vi "CRYAPI LOAD.vi"(4 "sTitle":string, 6 "sOption":string, 8 "sData":string, 9 "nData":i32, 10 "pSPRef":refnum<vi>, 11 "sAction":string) -> (0 "nData_Out":i32, 1 "tWindow_Out":T1, 2 "pVIRef_Out":refnum<vi>, 3 "pSPRef_Out":refnum<vi>)   [LabVIEW 2013]
uses:
  CRYMain Sub Window Global.vi
  DataView/VIEW/CRYView Global.vi
  CRYDocument/CRYReport Global.vi
  CRYProject/CRYProject Editor Global.vi
  CRYStepSetup/CRYStepSetup Global.vi
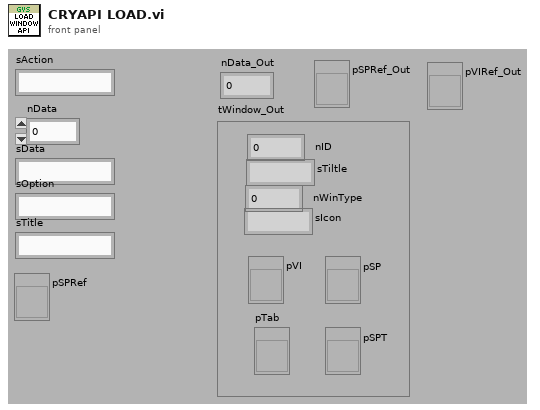
[diagram p1: front panel]
types:
  T1 = cluster{"nID":i32, "sTiltle":string, "pVI":refnum<vi>, "pSP":refnum<vi>, "pTab":refnum<vi>, "pSPT":refnum<vi>, "nWinType":i32, "sIcon":string}
  T2 = cluster{"sAction":string, "sType":string, "sQueueName":string, "sGraphName":string, "sData":string, "nData":i32, "pVIRef":refnum<vi>, "pSPRef":refnum<vi>}
  T3 = typedef "CRYTS.ctl" = cluster{"No.TS":u16, "TS File Path":path, "TS Name":string, "EditStepName":string, "Steps":T4[], "New State":bool, "Change State":bool, "Flattened CurveLib Data":string, "Document Data":string, "EditStepNo":u16, "Operator Start File":string, "Sequence Type":string, "Sequence Language":string}
  T4 = typedef "CRYStep.ctl" = cluster{"No.VI":i32, "Category":string, "StepName":string, "Seq setup flattened":string, "Comment":string, "Steps config.":bool[], "Jump config":i32[], "Start":dbl, "Increment":dbl, "Name":string, "Unit":string, "Y data":u16, "Y prefix":string, "Y dB ref":dbl, "Y unit":string, "Repeat State Array":cluster{"Start":dbl, "Increment":dbl, "Count":i32, "Num":i32}[]}
  T5 = cluster{"CLOSE_HIDE":i32, "CLOSE_CLOSE":i32, "DOCK_ENABLE":i32, "DOCK_DISABLE":i32, "FOCUS_SHOW":i32, "FOCUS_HIDE":i32}
  T6 = cluster{"sStepName":string, "nStepVINo":i32, "nStepVINoDisplay":i32}
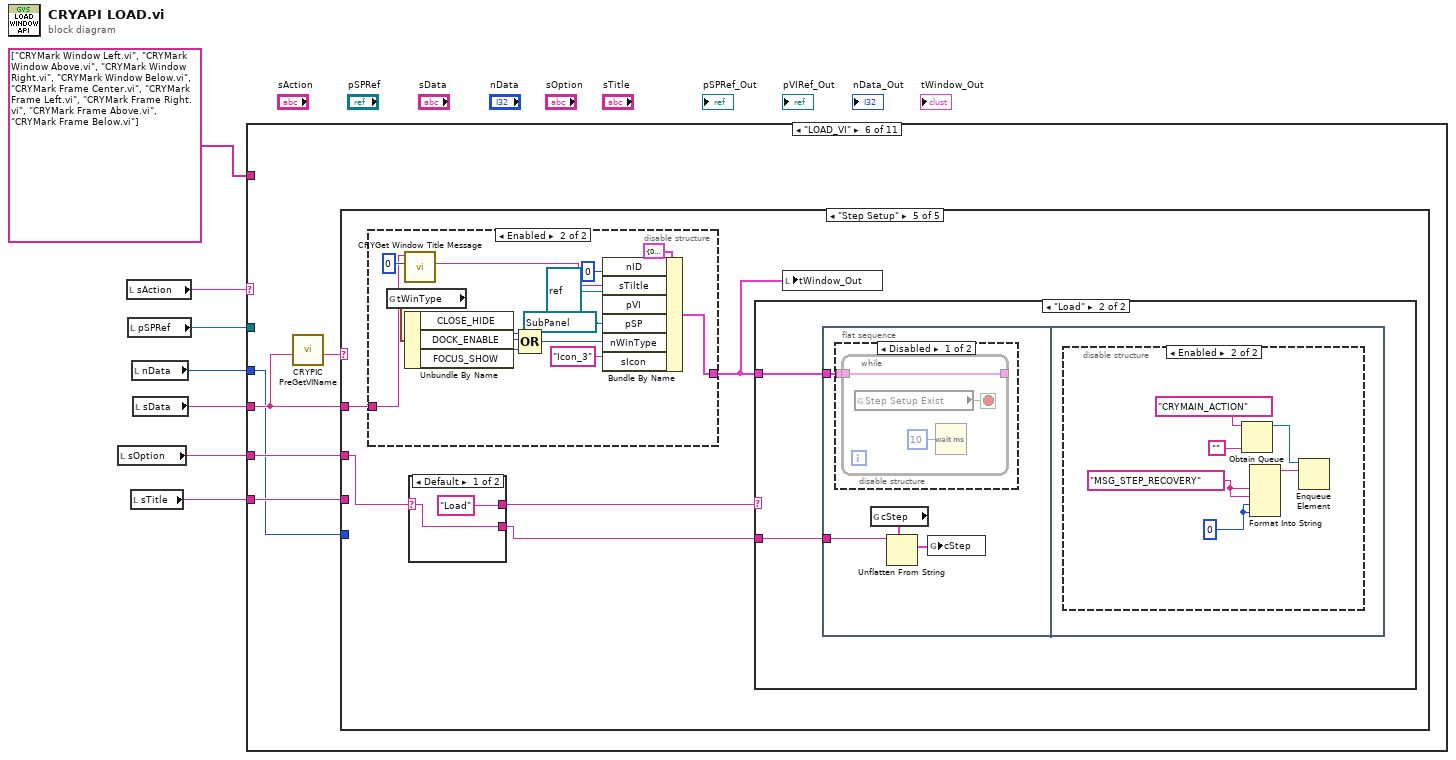
[diagram p0: block diagram]
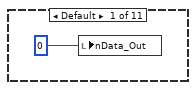
[diagram p2: hidden frame]
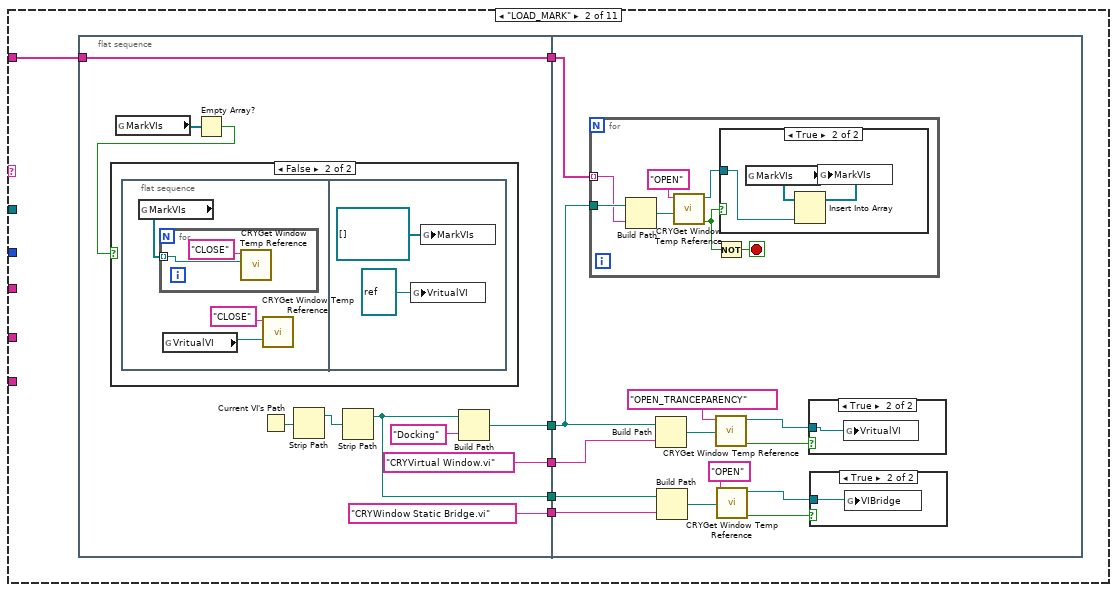
[diagram p3: hidden frame]
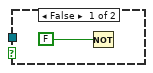
[diagram p5: hidden frame]
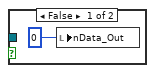
[diagram p6: hidden frame]
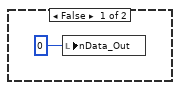
[diagram p7: hidden frame]
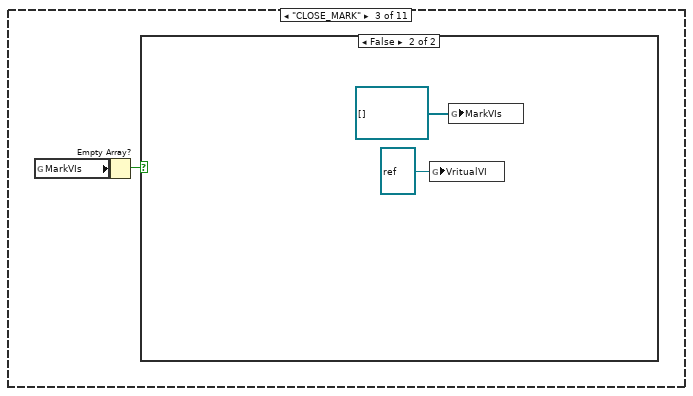
[diagram p8: hidden frame]
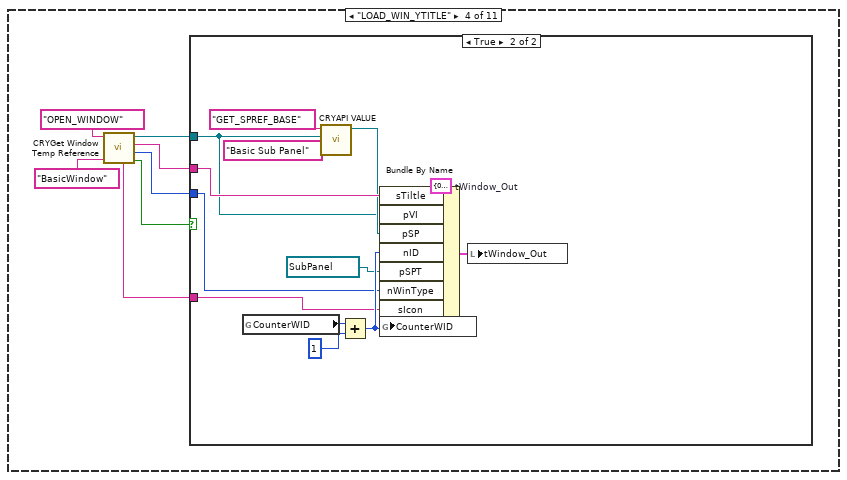
[diagram p10: hidden frame]
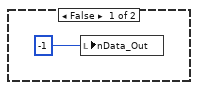
[diagram p11: hidden frame]
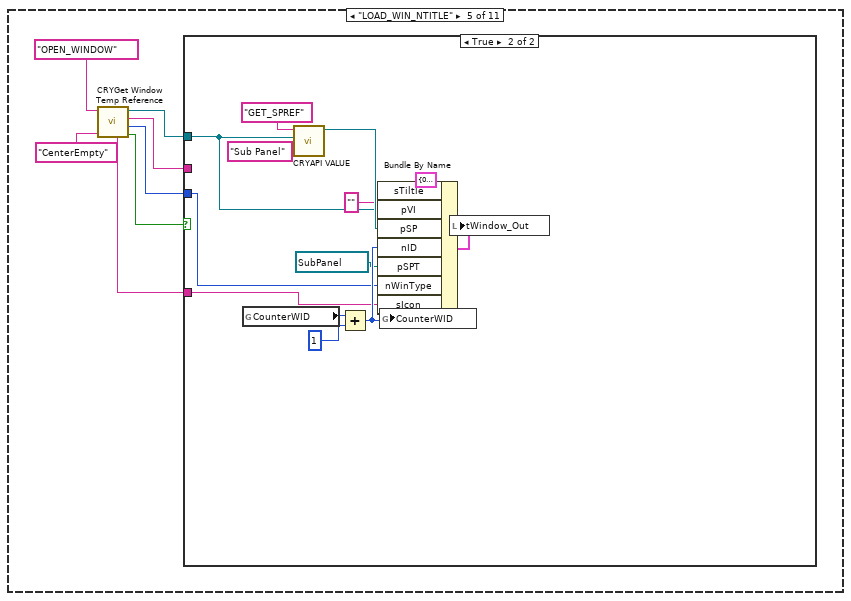
[diagram p12: hidden frame]
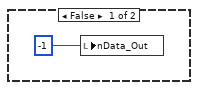
[diagram p13: hidden frame]
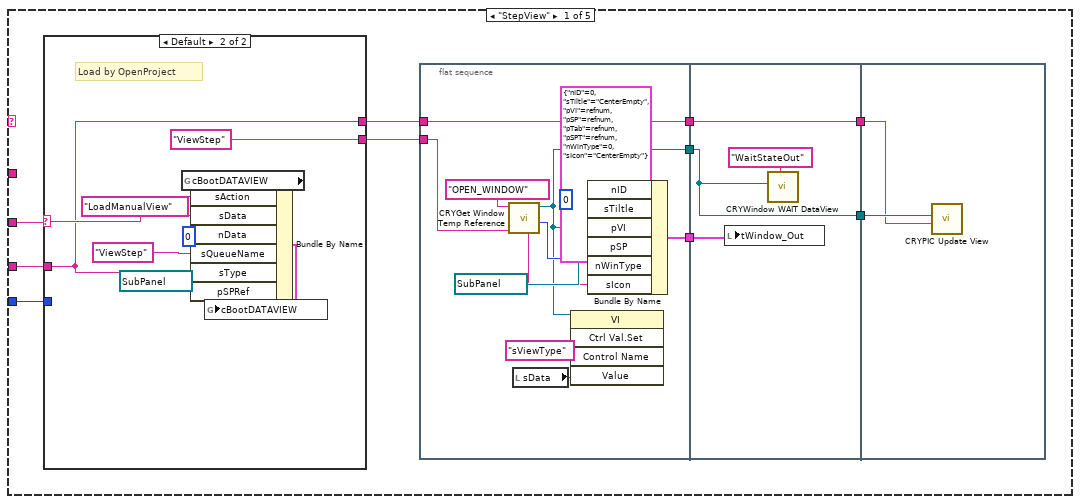
[diagram p14: hidden frame]
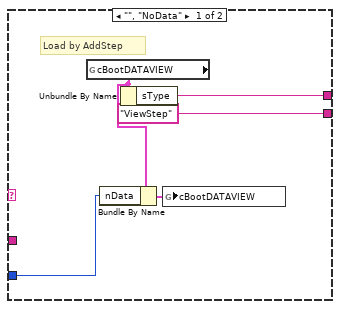
[diagram p15: hidden frame]
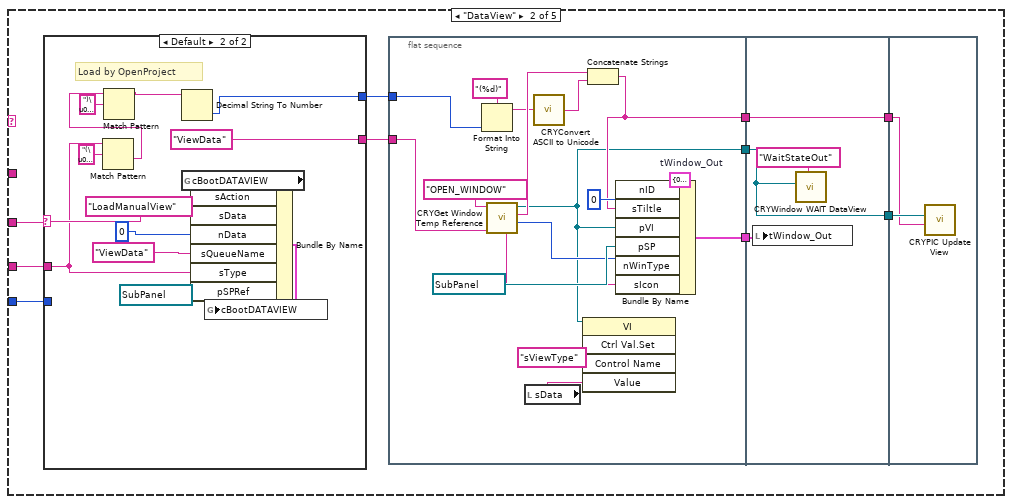
[diagram p16: hidden frame]
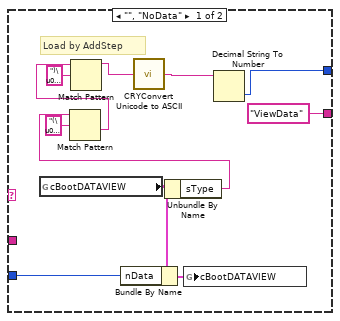
[diagram p17: hidden frame]
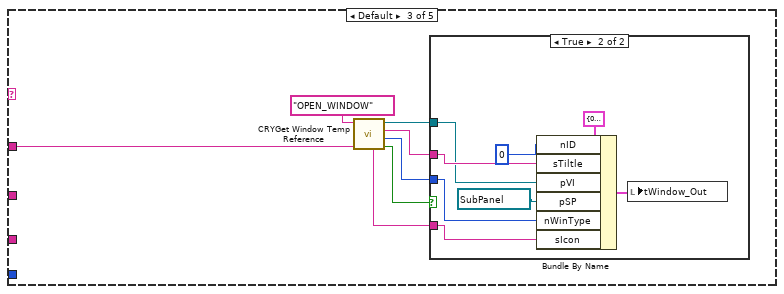
[diagram p18: hidden frame]
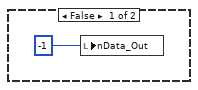
[diagram p19: hidden frame]
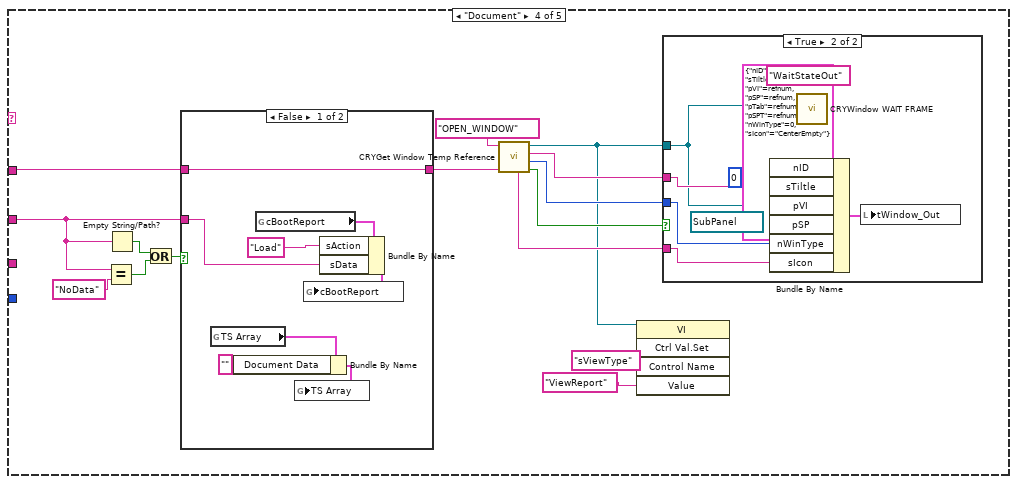
[diagram p20: hidden frame]
diagram:
  n1 = local read "sOption"() -> (w2:string)
  n2 = local read "sAction"() -> (w6:string)
  n3 = local read "pSPRef"() -> (w4:refnum<vi>)
  n4 = local read "sTitle"() -> (w1:string)
  n5 = local read "nData"() -> (w3:i32)
  n6 = local read "sData"() -> (w5:string)
  n7 = case shown="\"LOAD_VI\"" w6 {
    tunnel: string[] ["CRYMark Window Left.vi", "CRYMark Window Above.vi", "CRYMark Window Right.vi", "CRYMark Window Below.vi", "CRYMark Frame Center.vi", "CRYMark Frame Left.vi", "CRYMark Frame Right.vi", "CRYMark Frame Above.vi", "CRYMark Frame Below.vi"] -> [_ w13 _ _ _ _ _ _ _ _ _]
    tunnel: w5 -> [_ _ _ _ _ w107 _ w360 _ w395 _]
    tunnel: w4 -> [_ _ _ _ _ _ _ _ _ _ _]
    tunnel: w3 -> [_ _ _ _ _ w106 _ _ _ _ _]
    tunnel: w2 -> [_ _ _ _ _ w110 _ _ _ _ _]
    tunnel: w1 -> [_ _ _ _ _ w109 _ _ _ _ _]
    frame Default {
      n8 = local write "nData_Out"(0 ("nData_Out")) -> ()
    }
    frame "LOAD_MARK" {
      n9 = flat-sequence {
        tunnel: ["CRYVirtual Window.vi" ("name or relative path")] -> w14
        tunnel: w13 -> [w23]
        tunnel: [w23] -> w12
        tunnel: [w20] -> w11
        tunnel: [w16] -> w10
        tunnel: ["CRYWindow Static Bridge.vi" ("name or relative path")] -> w9
        tunnel: w14 -> [w38]
        tunnel: w12 -> [w43]
        tunnel: w11 -> [w40]
        tunnel: w10 -> [w33]
        tunnel: w9 -> [w32]
        frame #0 {
          n10 = global read "CRYMain Sub Window Global.vi" "MarkVIs"() -> (w19:refnum<vi>[])
          n11 = Empty Array?(array=w19) -> (empty?=w18:bool)
          n12 = case shown="False" w18 {
            frame True {
            }
            frame False {
              n13 = flat-sequence {
                frame #0 {
                  n14 = global read "CRYMain Sub Window Global.vi" "MarkVIs"() -> (w27:refnum<vi>[])
                  n15 = for {
                    tunnel: w27 -> [w28] mode=indexing
                    n16 = call "CRYGet Window Temp Reference.vi"("pVIRef_In"=w28, "sAction"="CLOSE") -> ()  [unwired: 2 in, 8 out]
                  }
                  n17 = global read "CRYMain Sub Window Global.vi" "VritualVI"() -> (w25:refnum<vi>)
                  n18 = call "CRYGet Window Temp Reference.vi"("pVIRef_In"=w25, "sAction"="CLOSE") -> ()  [unwired: 2 in, 8 out]
                }
                frame #1 {
                  n19 = global write "CRYMain Sub Window Global.vi" "VritualVI"(refnum<vi> refnum ("VIRef_Virtual")) -> ()
                  n20 = global write "CRYMain Sub Window Global.vi" "MarkVIs"(refnum<vi>[] [] ("VIRef_Mark")) -> ()
                }
              }
            }
          }
          n21 = Current VI's Path() -> (path=w22:path)
          n22 = Strip Path(path=w22) -> (stripped path=w21:path)  [unwired: 1 out]
          n23 = Strip Path(path=w21) -> (stripped path=w16:path)  [unwired: 1 out]
          n24 = Build Path(base path=w16, name or relative path="Docking") -> (appended path=w20:path)
        }
        frame #1 {
          n25 = for {
            tunnel: w40 -> [w55]
            tunnel: w43 -> [w54] mode=indexing
            stop <- w52 stop-if-true
            n26 = Build Path(base path=w55, name or relative path=w54) -> (appended path=w53:path)
            n27 = call "CRYGet Window Temp Reference.vi"("sVIFullName"=w53, "sAction"="OPEN") -> ("bResult"=w50:bool, "pVIRef_Out"=w49:refnum<vi>)  [unwired: 2 in, 6 out]
            n28 = Not(x=w50) -> (.not. x?=w52:bool)
            n29 = case shown="True" w50 {
              tunnel: w49 -> [_ w57]
              frame False {
                n30 = local write "nData_Out"(0 ("nData_Out")) -> ()
              }
              frame True {
                n31 = global read "CRYMain Sub Window Global.vi" "MarkVIs"() -> (w58:refnum<vi>[])
                n32 = Insert Into Array(array=w58, new element=w57) -> (w59:refnum<vi>[])  [unwired: 1 in]
                n33 = global write "CRYMain Sub Window Global.vi" "MarkVIs"(w59) -> ()
              }
            }
          }
          n34 = Build Path(base path=w40, name or relative path=w38) -> (appended path=w44:path)
          n35 = Build Path(base path=w33, name or relative path=w32) -> (appended path=w37:path)
          n36 = call "CRYGet Window Temp Reference.vi"("sVIFullName"=w44, "sAction"="OPEN_TRANCEPARENCY") -> ("bResult"=w41:bool, "pVIRef_Out"=w39:refnum<vi>)  [unwired: 2 in, 6 out]
          n37 = call "CRYGet Window Temp Reference.vi"("sVIFullName"=w37, "sAction"="OPEN") -> ("bResult"=w35:bool, "pVIRef_Out"=w34:refnum<vi>)  [unwired: 5 in, 3 out]
          n38 = case shown="True" w41 {
            tunnel: w39 -> [_ w48]
            frame False {
              n39 = local write "nData_Out"(0 ("nData_Out")) -> ()
            }
            frame True {
              n40 = global write "CRYMain Sub Window Global.vi" "VritualVI"(w48) -> ()
            }
          }
          n41 = case shown="True" w35 {
            tunnel: w34 -> [_ w46]
            frame False {
              n42 = Not(x=FALSE) -> ()  [unwired: 1 out]
            }
            frame True {
              n43 = global write "CRYMain Sub Window Global.vi" "VIBridge"(w46) -> ()
            }
          }
        }
      }
    }
    frame "CLOSE_MARK" {
      n44 = global read "CRYMain Sub Window Global.vi" "MarkVIs"() -> (w60:refnum<vi>[])
      n45 = Empty Array?(array=w60) -> (empty?=w61:bool)
      n46 = case shown="False" w61 {
        frame True {
        }
        frame False {
          n47 = global write "CRYMain Sub Window Global.vi" "VritualVI"(refnum<vi> refnum ("VIRef_Virtual")) -> ()
          n48 = global write "CRYMain Sub Window Global.vi" "MarkVIs"(refnum<vi>[] [] ("VIRef_Mark")) -> ()
        }
      }
    }
    frame "LOAD_WIN_YTITLE" {
      n49 = call "CRYGet Window Temp Reference.vi"("sWindowName"="BasicWindow", "sAction"="OPEN_WINDOW") -> ("bResult"=w65:bool, "nWinType"=w70:i32, "sTitleName Out"=w69:string, "pVIRef_Out"=w66:refnum<vi>, "sIcon_Out"=w64:string)  [unwired: 2 in, 3 out]
      n50 = case shown="True" w65 {
        tunnel: w66 -> [_ w77]
        tunnel: w69 -> [_ w79]
        tunnel: w70 -> [_ w74]
        tunnel: w64 -> [_ w72]
        frame False {
          n51 = local write "nData_Out"(-1 ("nData_Out")) -> ()
        }
        frame True {
          w73 = T1 {"nID"=0, "sTiltle"="CenterEmpty", "pVI"=refnum, "pSP"=refnum, "pTab"=refnum, "pSPT"=refnum, "nWinType"=0, "sIcon"="CenterEmpty"}  # tWindow_Out
          n52 = global read "CRYMain Sub Window Global.vi" "CounterWID"() -> (w84:i32)
          n53 = call "CRYAPI VALUE.vi"("sControlName"="Basic Sub Panel", "pVIRef"=w77, "sAction"="GET_SPREF_BASE") -> ("pSPRef"=w78:refnum<vi>)  [unwired: 2 in, 6 out]
          n54 = Add(x=w84, y=1) -> (x+y=w76:i32)
          n55 = Bundle By Name(cluster=w73, "sTiltle"=w79, "pVI"=w77, "pSP"=w78, "nID"=w76, "pSPT"=refnum<vi> refnum, "nWinType"=w74, "sIcon"=w72) -> (w80:T1)
          n56 = global write "CRYMain Sub Window Global.vi" "CounterWID"(w76) -> ()
          n57 = local write "tWindow_Out"(w80) -> ()
        }
      }
    }
    frame "LOAD_WIN_NTITLE" {
      n58 = call "CRYGet Window Temp Reference.vi"("sWindowName"="CenterEmpty", "sAction"="OPEN_WINDOW") -> ("bResult"=w86:bool, "nWinType"=w91:i32, "sTitleName Out"=w90:string, "pVIRef_Out"=w87:refnum<vi>, "sIcon_Out"=w85:string)  [unwired: 2 in, 3 out]
      n59 = case shown="True" w86 {
        tunnel: w87 -> [_ w98]
        tunnel: w90 -> [_ _]
        tunnel: w91 -> [_ w95]
        tunnel: w85 -> [_ w93]
        frame False {
          n60 = local write "nData_Out"(-1 ("nData_Out")) -> ()
        }
        frame True {
          n61 = global read "CRYMain Sub Window Global.vi" "CounterWID"() -> (w100:i32)
          n62 = call "CRYAPI VALUE.vi"("sControlName"="Sub Panel", "pVIRef"=w98, "sAction"="GET_SPREF") -> ("pSPRef"=w99:refnum<vi>)  [unwired: 2 in, 6 out]
          n63 = Add(x=w100, y=1) -> (x+y=w103:i32)
          n64 = Bundle By Name(cluster=T1 {"nID"=0, "sTiltle"="CenterEmpty", "pVI"=refnum, "pSP"=refnum, "pTab"=refnum, "pSPT"=refnum, "nWinType"=0, "sIcon"="CenterEmpty"} ("tWindow_Out"), "sTiltle"="", "pVI"=w98, "pSP"=w99, "nID"=w103, "pSPT"=refnum<vi> refnum, "nWinType"=w95, "sIcon"=w93) -> (w102:T1)
          n65 = global write "CRYMain Sub Window Global.vi" "CounterWID"(w103) -> ()
          n66 = local write "tWindow_Out"(w102) -> ()
        }
      }
    }
    frame "LOAD_VI" {
      n67 = call "CRYPIC PreGetVIName.vi"("sVIName"=w107) -> ("sVIName_Out"=w108:string)  [unwired: 9 in, 1 out]
      n68 = case shown="\"Step Setup\"" w108 {
        tunnel: w107 -> [_ _ w212 w236 w265]
        tunnel: w110 -> [w118 w158 _ w234 w268]
        tunnel: w109 -> [w117 w157 _ _ _]
        tunnel: w106 -> [w111 w153 _ _ _]
        frame "StepView" {
          n69 = case shown="Default" w118 {
            selector: w118 -> [_ w147]
            tunnel: ["ViewStep" ("sData") "ViewStep" ("sData")] -> w120
            tunnel: [w142 w146] -> w119
            tunnel: w117 -> [_ w146]
            tunnel: w111 -> [w139 _]
            frame "", "NoData" {
              # "Load by AddStep"
              n70 = global read "CRYView Global.vi" "cBootDATAVIEW"() -> (w140:T2)
              n71 = Bundle By Name(cluster=w140, "nData"=w139) -> (w141:T2)
              n72 = Unbundle By Name(w140) -> ("sType"=w142:string)
              n73 = global write "CRYView Global.vi" "cBootDATAVIEW"(w141) -> ()
            }
            frame Default {
              # "Load by OpenProject"
              n74 = global read "CRYView Global.vi" "cBootDATAVIEW"() -> (w148:T2)
              n75 = Bundle By Name(cluster=w148, "sAction"="LoadManualView" ("sData"), "sData"=w147, "nData"=0, "sQueueName"="ViewStep" ("sData"), "sType"=w146, "pSPRef"=refnum<vi> refnum) -> (w149:T2)
              n76 = global write "CRYView Global.vi" "cBootDATAVIEW"(w149) -> ()
            }
          }
          n77 = flat-sequence {
            tunnel: [w126] -> w116
            tunnel: [w122] -> w115
            tunnel: w119 -> [w125]
            tunnel: w120 -> [w123]
            tunnel: [w125] -> w114
            tunnel: w116 -> [w136]
            tunnel: w115 -> [w134]
            tunnel: [w134] -> w113
            tunnel: [w133] -> w112
            tunnel: w114 -> [w133]
            tunnel: w113 -> [w138]
            tunnel: w112 -> [w137]
            frame #0 {
              n78 = call "CRYGet Window Temp Reference.vi"("sWindowName"=w123, "sAction"="OPEN_WINDOW") -> ("nWinType"=w127:i32, "pVIRef_Out"=w122:refnum<vi>, "sIcon_Out"=w129:string)  [unwired: 2 in, 5 out]
              n79 = local read "sData"() -> (w121:string)
              n80 = invoke class="VI" method="Ctrl Val.Set"(reference=w122, "Control Name"="sViewType", "Value"=w121) -> ()  [unwired: 2 in, 5 out]
              n81 = Bundle By Name(cluster=T1 {"nID"=0, "sTiltle"="CenterEmpty", "pVI"=refnum, "pSP"=refnum, "pTab"=refnum, "pSPT"=refnum, "nWinType"=0, "sIcon"="CenterEmpty"} ("tWindow_Out"), "nID"=0, "sTiltle"=w125, "pVI"=w122, "pSP"=refnum<vi> refnum ("pSPRef"), "nWinType"=w127, "sIcon"=w129) -> (w126:T1)
            }
            frame #1 {
              n82 = local write "tWindow_Out"(w136) -> ()
              n83 = call "CRYWindow WAIT DataView.vi"("vi reference"=w134, "sAction"="WaitStateOut") -> ()  [unwired: 9 in, 1 out]
            }
            frame #2 {
              n84 = call "CRYPIC Update View.vi"("sTitle"=w137, "pVIRef"=w138) -> ()  [unwired: 10 in]
            }
          }
        }
        frame "DataView" {
          n85 = case shown="Default" w158 {
            selector: w158 -> [_ w182]
            tunnel: ["ViewData" ("sData") "ViewData" ("sData")] -> w160
            tunnel: w157 -> [_ w179]
            tunnel: [w168 w177] -> w156
            tunnel: w153 -> [w163 _]
            frame "", "NoData" {
              # "Load by AddStep"
              n86 = global read "CRYView Global.vi" "cBootDATAVIEW"() -> (w165:T2)
              n87 = Bundle By Name(cluster=w165, "nData"=w163) -> (w164:T2)
              n88 = Unbundle By Name(w165) -> ("sType"=w169:string)
              n89 = Match Pattern(string=w169, regular expression="(\u0000") -> (after substring=w170:string)  [unwired: 1 in, 3 out]
              n90 = Match Pattern(string=w170, regular expression=")\u0000") -> (before substring=w166:string)  [unwired: 1 in, 3 out]
              n91 = call "CRYConvert Unicode to ASCII.vi"("Unicode"=w166) -> ("ASCII"=w167:string)  [unwired: 4 in]
              n92 = global write "CRYView Global.vi" "cBootDATAVIEW"(w164) -> ()
              n93 = Decimal String To Number(string=w167) -> (number=w168:i32)  [unwired: 2 in, 1 out]
            }
            frame Default {
              # "Load by OpenProject"
              n94 = Match Pattern(string=w179, regular expression="(\u0000") -> (after substring=w178:string)  [unwired: 1 in, 3 out]
              n95 = Match Pattern(string=w178, regular expression=")\u0000") -> (before substring=w176:string)  [unwired: 1 in, 3 out]
              n96 = Decimal String To Number(string=w176) -> (number=w177:i32)  [unwired: 2 in, 1 out]
              n97 = global read "CRYView Global.vi" "cBootDATAVIEW"() -> (w183:T2)
              n98 = Bundle By Name(cluster=w183, "sAction"="LoadManualView" ("sData"), "sData"=w182, "nData"=0, "sQueueName"="ViewData" ("sData"), "sType"=w179, "pSPRef"=refnum<vi> refnum) -> (w184:T2)
              n99 = global write "CRYView Global.vi" "cBootDATAVIEW"(w184) -> ()
            }
          }
          n100 = flat-sequence {
            tunnel: [w198] -> w162
            tunnel: [w191] -> w161
            tunnel: w160 -> [w190]
            tunnel: w156 -> [w197]
            tunnel: [w192] -> w154
            tunnel: w162 -> [w208]
            tunnel: w161 -> [w206]
            tunnel: [w206] -> w159
            tunnel: [w205] -> w155
            tunnel: w154 -> [w205]
            tunnel: w159 -> [w210]
            tunnel: w155 -> [w209]
            frame #0 {
              w204 = T1 {"nID"=0, "sTiltle"="CenterEmpty", "pVI"=refnum, "pSP"=refnum, "pTab"=refnum, "pSPT"=refnum, "nWinType"=0, "sIcon"="CenterEmpty"}  # tWindow_Out
              n101 = Format Into String(format string="(%d)", w197) -> (resulting string=w194:string)  [unwired: 2 in, 1 out]
              n102 = call "CRYGet Window Temp Reference.vi"("sWindowName"=w190, "sAction"="OPEN_WINDOW") -> ("nWinType"=w199:i32, "sTitleName Out"=w196:string, "pVIRef_Out"=w191:refnum<vi>, "sIcon_Out"=w201:string)  [unwired: 2 in, 4 out]
              n103 = local read "sData"() -> (w188:string)
              n104 = call "CRYConvert ASCII to Unicode.vi"("ASCII"=w194) -> ("Unicode"=w193:string)  [unwired: 4 in]
              n105 = invoke class="VI" method="Ctrl Val.Set"(reference=w191, "Control Name"="sViewType", "Value"=w188) -> ()  [unwired: 2 in, 5 out]
              n106 = Concatenate Strings(w196, w193) -> (w192:string)
              n107 = Bundle By Name(cluster=w204, "nID"=0, "sTiltle"=w192, "pVI"=w191, "pSP"=refnum<vi> refnum ("pSPRef"), "nWinType"=w199, "sIcon"=w201) -> (w198:T1)
            }
            frame #1 {
              n108 = local write "tWindow_Out"(w208) -> ()
              n109 = call "CRYWindow WAIT DataView.vi"("vi reference"=w206, "sAction"="WaitStateOut") -> ()  [unwired: 9 in, 1 out]
            }
            frame #2 {
              n110 = call "CRYPIC Update View.vi"("sTitle"=w209, "pVIRef"=w210) -> ()  [unwired: 10 in]
            }
          }
        }
        frame Default {
          n111 = call "CRYGet Window Temp Reference.vi"("sWindowName"=w212, "sAction"="OPEN_WINDOW") -> ("bResult"=w215:bool, "nWinType"=w217:i32, "sTitleName Out"=w216:string, "pVIRef_Out"=w213:refnum<vi>, "sIcon_Out"=w211:string)  [unwired: 2 in, 3 out]
          n112 = case shown="True" w215 {
            tunnel: w213 -> [_ w224]
            tunnel: w216 -> [_ w225]
            tunnel: w217 -> [_ w222]
            tunnel: w211 -> [_ w220]
            frame False {
              n113 = local write "nData_Out"(-1 ("nData_Out")) -> ()
            }
            frame True {
              n114 = Bundle By Name(cluster=T1 {"nID"=0, "sTiltle"="CenterEmpty", "pVI"=refnum, "pSP"=refnum, "pTab"=refnum, "pSPT"=refnum, "nWinType"=0, "sIcon"="CenterEmpty"} ("tWindow_Out"), "nID"=0, "sTiltle"=w225, "pVI"=w224, "pSP"=refnum<vi> refnum ("pSPRef"), "nWinType"=w222, "sIcon"=w220) -> (w219:T1)
              n115 = local write "tWindow_Out"(w219) -> ()
            }
          }
        }
        frame "Document" {
          n116 = Equal?(x=w234, y="NoData") -> (x = y?=w230:bool)
          n117 = Empty String/Path?(string/path=w234) -> (empty?=w231:bool)
          n118 = Or(x=w231, y=w230) -> (x .or. y?=w232:bool)
          n119 = case shown="False" w232 {
            tunnel: w234 -> [w246 _]
            tunnel: w236 -> [w245 w250]
            tunnel: [w245 w250] -> w235
            frame False {
              n120 = global read "CRYProject Editor Global.vi" "TS Array"() -> (w244:T3)
              n121 = Bundle By Name(cluster=w244, "Document Data"="") -> (w242:T3)
              n122 = global read "CRYReport Global.vi" "cBootReport"() -> (w247:T2)
              n123 = global write "CRYProject Editor Global.vi" "TS Array"(w242) -> ()
              n124 = Bundle By Name(cluster=w247, "sAction"="Load", "sData"=w246) -> (w249:T2)
              n125 = global write "CRYReport Global.vi" "cBootReport"(w249) -> ()
            }
            frame True {
              n126 = global read "CRYReport Global.vi" "cBootReport"() -> (w251:T2)
              n127 = Bundle By Name(cluster=w251, "sAction"="New", "sData"="") -> (w253:T2)
              n128 = global write "CRYReport Global.vi" "cBootReport"(w253) -> ()
            }
          }
          n129 = call "CRYGet Window Temp Reference.vi"("sWindowName"=w235, "sAction"="OPEN_WINDOW") -> ("bResult"=w239:bool, "nWinType"=w241:i32, "sTitleName Out"=w240:string, "pVIRef_Out"=w228:refnum<vi>, "sIcon_Out"=w237:string)  [unwired: 2 in, 3 out]
          n130 = invoke class="VI" method="Ctrl Val.Set"(reference=w228, "Control Name"="sViewType", "Value"="ViewReport" ("Control Name")) -> ()  [unwired: 2 in, 5 out]
          n131 = case shown="True" w239 {
            tunnel: w228 -> [_ w256]
            tunnel: w240 -> [_ w263]
            tunnel: w241 -> [_ w261]
            tunnel: w237 -> [_ w259]
            frame False {
              n132 = local write "nData_Out"(-1 ("nData_Out")) -> ()
            }
            frame True {
              n133 = Bundle By Name(cluster=T1 {"nID"=0, "sTiltle"="CenterEmpty", "pVI"=refnum, "pSP"=refnum, "pTab"=refnum, "pSPT"=refnum, "nWinType"=0, "sIcon"="CenterEmpty"} ("tWindow_Out"), "nID"=0, "sTiltle"=w263, "pVI"=w256, "pSP"=refnum<vi> refnum ("pSPRef"), "nWinType"=w261, "sIcon"=w259) -> (w258:T1)
              n134 = call "CRYWindow WAIT FRAME.vi"("sAction"="WaitStateOut", "vi reference"=w256) -> ()  [unwired: 9 in, 1 out]
              n135 = local write "tWindow_Out"(w258) -> ()
            }
          }
        }
        frame "Step Setup" {
          n136 = disable-structure shown="Enabled" {
            disable-tunnel: [w271 w288] -> w269
            disable-tunnel: w265 -> [w270 w300]
            frame Disabled {
              n137 = call "CRYGet Window Temp Reference.vi"("sWindowName"=w270, "sAction"="OPEN_WINDOW") -> ("bResult"=w275:bool, "nWinType"=w277:i32, "sTitleName Out"=w276:string, "pVIRef_Out"=w273:refnum<vi>, "sIcon_Out"=w272:string)  [unwired: 2 in, 3 out]
              n138 = case shown="True" w275 {
                tunnel: w273 -> [_ w285]
                tunnel: w276 -> [_ w286]
                tunnel: w277 -> [_ w283]
                tunnel: w272 -> [_ w281]
                tunnel: [T1 {"nID"=0, "sTiltle"="", "pVI"=refnum, "pSP"=refnum, "pTab"=refnum, "pSPT"=refnum, "nWinType"=0, "sIcon"=""} ("tWindow_Out") w280] -> w271
                frame False {
                  n139 = local write "nData_Out"(-1 ("nData_Out")) -> ()
                }
                frame True {
                  n140 = Bundle By Name(cluster=T1 {"nID"=0, "sTiltle"="CenterEmpty", "pVI"=refnum, "pSP"=refnum, "pTab"=refnum, "pSPT"=refnum, "nWinType"=0, "sIcon"="CenterEmpty"} ("tWindow_Out"), "nID"=0, "sTiltle"=w286, "pVI"=w285, "pSP"=refnum<vi> refnum ("pSPRef"), "nWinType"=w283, "sIcon"=w281) -> (w280:T1)
                }
              }
            }
            frame Enabled {
              n141 = global read "CRYMain Sub Window Global.vi" "tWinType"() -> (w298:T5)
              n142 = call "CRYGet Window Title Message.vi"("No"=0 ("Error No"), "Kind"=w300) -> ("Unicode String"=w290:string)  [unwired: 4 in, 5 out]
              n143 = Unbundle By Name(w298) -> ("CLOSE_HIDE"=w297:i32, "DOCK_ENABLE"=w296:i32, "FOCUS_SHOW"=w295:i32)
              n144 = Compound Arithmetic op=OR(w297, w296, w295) -> (w299:i32)
              n145 = Bundle By Name(cluster=T1 {"nID"=0, "sTiltle"="CenterEmpty", "pVI"=refnum, "pSP"=refnum, "pTab"=refnum, "pSPT"=refnum, "nWinType"=0, "sIcon"="CenterEmpty"} ("tWindow_Out"), "nID"=0, "sTiltle"=w290, "pVI"=refnum<vi> refnum, "pSP"=refnum<vi> refnum, "nWinType"=w299, "sIcon"="Icon_3") -> (w288:T1)
            }
          }
          n146 = case shown="Default" w268 {
            selector: w268 -> [w302 _]
            tunnel: ["Load" ("sData") "New" ("sData")] -> w267
            tunnel: [w302 "" ("sData")] -> w266
            frame Default {
            }
            frame "NoData" {
            }
          }
          n147 = case shown="\"Load\"" w267 {
            tunnel: w266 -> [_ w306]
            tunnel: w269 -> [_ w307]
            frame "False", Default {
            }
            frame "Load" {
              n148 = flat-sequence {
                tunnel: w307 -> [w311]
                tunnel: w306 -> [w310]
                frame #0 {
                  n149 = disable-structure shown="Disabled" {
                    disable-tunnel: w311 -> [w312 _]
                    frame Disabled {
                      n150 = while {
                        tunnel: w312 -> [w313]
                        tunnel: [w313] -> _
                        stop <- w315 stop-if-true
                        n151 = global read "CRYStepSetup Global.vi" "Step Setup Exist"() -> (w315:bool)
                        n152 = Wait (ms)(milliseconds to wait=u32 10) -> ()  [unwired: 1 out]
                      }
                    }
                    frame Enabled {
                    }
                  }
                  n153 = global read "CRYStepSetup Global.vi" "cStep"() -> (w309:T6)
                  n154 = Unflatten From String(type=w309, binary string=w310) -> (value=w308:T6)  [unwired: 1 in, 4 out]
                  n155 = global write "CRYStepSetup Global.vi" "cStep"(w308) -> ()
                }
                frame #1 {
                  n156 = disable-structure shown="Enabled" {
                    frame Disabled {
                      n157 = global read "CRYMain Sub Window Global.vi" "MsgProVI"() -> (w317:refnum<vi>)
                      n158 = call "CRYGet Boolean Reference.vi"("Label Name"="bStepRecovery", "VI Refnum"=w317) -> ("Exist?"=w318:bool, "Boolean Ref"=w319:refnum<vi>)  [unwired: 7 in, 1 out]
                      n159 = case shown="True" w318 {
                        tunnel: w319 -> [_ w320]
                        frame False {
                        }
                        frame True {
                          n160 = property class="Bool"(reference=w320, "Val(Sgnl)"=FALSE) -> ()  [unwired: 1 in, 2 out]
                        }
                      }
                    }
                    frame Enabled {
                      w322 = 0 ("input 3")
                      w327 = "MSG_STEP_RECOVERY" ("input 1")
                      n161 = Obtain Queue(name (unnamed)="CRYMAIN_ACTION" ("YAxisTitle"), element data type="" ("Action Type")) -> (queue out=w326:refnum<queue>)  [unwired: 3 in, 2 out]
                      n162 = Format Into String(w327, w327, w322, w322) -> (resulting string=w325:string)  [unwired: 3 in, 1 out]
                      n163 = Enqueue Element(queue=w326, element=w325) -> ()  [unwired: 1 in, 4 out]
                    }
                  }
                }
              }
            }
          }
          n164 = local write "tWindow_Out"(w269) -> ()
        }
      }
    }
    frame "LOAD_TAB" {
      n165 = call "CRYGet Window Temp Reference.vi"("sWindowName"="TAB", "sAction"="OPEN_WINDOW") -> ("bResult"=w332:bool, "nWinType"=w334:i32, "sTitleName Out"=w333:string, "pVIRef_Out"=w330:refnum<vi>, "sIcon_Out"=w328:string)  [unwired: 2 in, 3 out]
      n166 = case shown="True" w332 {
        tunnel: w330 -> [_ w336]
        tunnel: w333 -> [_ w350]
        tunnel: w334 -> [_ w341]
        tunnel: w328 -> [_ w339]
        frame False {
          n167 = local write "nData_Out"(-1 ("nData_Out")) -> ()
        }
        frame True {
          n168 = call "CRYAPI TAB Get Tab Reference.vi"("Label Name"="Tab Control", "VI Refnum"=w336) -> ("Tab Control Ref"=w348:refnum<vi>)  [unwired: 9 out]
          n169 = call "CRYAPI VALUE.vi"("sControlName"="Sub Panel", "pVIRef"=w336, "sAction"="GET_SPREF") -> ("pSPRef"=w345:refnum<vi>)  [unwired: 2 in, 6 out]
          n170 = call "CRYAPI VALUE.vi"("sControlName"="Sub Panel Next", "pVIRef"=w336, "sAction"="GET_SPREF") -> ("pSPRef"=w343:refnum<vi>)  [unwired: 2 in, 6 out]
          n171 = Bundle By Name(cluster=T1 {"nID"=0, "sTiltle"="CenterEmpty", "pVI"=refnum, "pSP"=refnum, "pTab"=refnum, "pSPT"=refnum, "nWinType"=0, "sIcon"="CenterEmpty"} ("tWindow_Out"), "nID"=0, "sTiltle"=w350, "pVI"=w336, "pSP"=w345, "pTab"=w348, "pSPT"=w343, "nWinType"=w341, "sIcon"=w339) -> (w338:T1)
          n172 = while {
            tunnel: [w357] -> w337
            tunnel: w338 -> [w357]
            tunnel: w336 -> [w356]
            stop <- w353 stop-if-true
            n173 = invoke class="VI" method="Ctrl Val.Get"(reference=w356, "Control Name"="StateOut") -> ("Get Control Value Variant"=w354:variant)  [unwired: 2 in, 3 out]
            n174 = Wait (ms)(milliseconds to wait=u32 10) -> ()  [unwired: 1 out]
            n175 = Variant To Data(type=TRUE, Variant=w354) -> (data=w353:bool)  [unwired: 1 in, 1 out]
          }
          n176 = local write "tWindow_Out"(w337) -> ()
        }
      }
    }
    frame "LOAD_SPLITER" {
      n177 = call "CRYGet Window Temp Reference.vi"("sWindowName"=w360, "sAction"="OPEN_WINDOW") -> ("bResult"=w363:bool, "nWinType"=w365:i32, "sTitleName Out"=w364:string, "pVIRef_Out"=w361:refnum<vi>, "sIcon_Out"=w359:string)  [unwired: 2 in, 3 out]
      n178 = case shown="True" w363 {
        tunnel: w361 -> [_ w374]
        tunnel: w364 -> [_ w375]
        tunnel: w365 -> [_ _]
        tunnel: w359 -> [_ w367]
        frame False {
          n179 = local write "nData_Out"(-1 ("nData_Out")) -> ()
        }
        frame True {
          n180 = global read "CRYMain Sub Window Global.vi" "CounterSpliter"() -> (w370:i32)
          n181 = Subtract(x=w370, y=1) -> (x-y=w369:i32)
          n182 = Bundle By Name(cluster=T1 {"nID"=0, "sTiltle"="CenterEmpty", "pVI"=refnum, "pSP"=refnum, "pTab"=refnum, "pSPT"=refnum, "nWinType"=0, "sIcon"="CenterEmpty"} ("tWindow_Out"), "sTiltle"=w375, "pVI"=w374, "pSP"=refnum<vi> refnum ("pSPRef"), "nID"=w369, "sIcon"=w367) -> (w372:T1)
          n183 = global write "CRYMain Sub Window Global.vi" "CounterSpliter"(w369) -> ()
          n184 = local write "tWindow_Out"(w372) -> ()
        }
      }
    }
    frame "LOAD_EMPTY" {
      n185 = call "CRYGet Window Temp Reference.vi"("sWindowName"="CenterEmpty", "sAction"="OPEN_WINDOW") -> ("bResult"=w380:bool, "nWinType"=w382:i32, "sTitleName Out"=w381:string, "pVIRef_Out"=w378:refnum<vi>, "sIcon_Out"=w376:string)  [unwired: 2 in, 3 out]
      n186 = case shown="True" w380 {
        tunnel: w378 -> [_ w389]
        tunnel: w381 -> [_ w390]
        tunnel: w382 -> [_ w386]
        tunnel: w376 -> [_ w384]
        frame False {
          n187 = local write "nData_Out"(0 ("nData_Out")) -> ()
        }
        frame True {
          w385 = T1 {"nID"=0, "sTiltle"="CenterEmpty", "pVI"=refnum, "pSP"=refnum, "pTab"=refnum, "pSPT"=refnum, "nWinType"=0, "sIcon"="CenterEmpty"}  # tWindow_Out
          n188 = call "CRYAPI VALUE.vi"("sControlName"="Sub Panel", "pVIRef"=w389, "sAction"="GET_SPREF") -> ("pSPRef"=w391:refnum<vi>)  [unwired: 2 in, 6 out]
          n189 = Bundle By Name(cluster=w385, "sTiltle"=w390, "pVI"=w389, "pSP"=w391, "nID"=0, "pSPT"=refnum<vi> refnum, "nWinType"=w386, "sIcon"=w384) -> (w392:T1)
          n190 = local write "tWindow_Out"(w392) -> ()
        }
      }
    }
    frame "LOAD_SUBPANEL" {
      n191 = call "CRYGet Window Temp Reference.vi"("sWindowName"=w395, "sAction"="OPEN_WINDOW") -> ("bResult"=w399:bool, "nWinType"=w401:i32, "sTitleName Out"=w400:string, "pVIRef_Out"=w397:refnum<vi>, "sIcon_Out"=w396:string)  [unwired: 2 in, 3 out]
      n192 = case shown="True" w399 {
        tunnel: w397 -> [_ w408]
        tunnel: w400 -> [_ w409]
        tunnel: w401 -> [_ w405]
        tunnel: w396 -> [_ w403]
        frame False {
          n193 = local write "nData_Out"(0 ("nData_Out")) -> ()
        }
        frame True {
          n194 = call "CRYAPI VALUE.vi"("sControlName"="Sub Panel", "pVIRef"=w408, "sAction"="GET_SPREF") -> ("pSPRef"=w410:refnum<vi>)  [unwired: 2 in, 6 out]
          n195 = Bundle By Name(cluster=T1 {"nID"=0, "sTiltle"="CenterEmpty", "pVI"=refnum, "pSP"=refnum, "pTab"=refnum, "pSPT"=refnum, "nWinType"=0, "sIcon"="CenterEmpty"} ("tWindow_Out"), "sTiltle"=w409, "pVI"=w408, "pSP"=w410, "nID"=0, "pSPT"=refnum<vi> refnum, "nWinType"=w405, "sIcon"=w403) -> (w411:T1)
          n196 = local write "tWindow_Out"(w411) -> ()
        }
      }
    }
    frame "LOAD_MSGPRO" {
      n197 = call "CRYGet Window Temp Reference.vi"("sWindowName"="MsgProcesser", "sAction"="OPEN_WINDOW") -> ("bResult"=w418:bool, "nWinType"=w420:i32, "sTitleName Out"=w419:string, "pVIRef_Out"=w416:refnum<vi>, "sIcon_Out"=w414:string)  [unwired: 2 in, 3 out]
      n198 = case shown="True" w418 {
        tunnel: w416 -> [_ w427]
        tunnel: w419 -> [_ w428]
        tunnel: w420 -> [_ w424]
        tunnel: w414 -> [_ w422]
        frame False {
          n199 = local write "nData_Out"(0 ("nData_Out")) -> ()
        }
        frame True {
          n200 = call "CRYAPI VALUE.vi"("sControlName"="Sub Panel", "pVIRef"=w427, "sAction"="GET_SPREF") -> ("pSPRef"=w429:refnum<vi>)  [unwired: 2 in, 6 out]
          n201 = Bundle By Name(cluster=T1 {"nID"=0, "sTiltle"="CenterEmpty", "pVI"=refnum, "pSP"=refnum, "pTab"=refnum, "pSPT"=refnum, "nWinType"=0, "sIcon"="CenterEmpty"} ("tWindow_Out"), "sTiltle"=w428, "pVI"=w427, "pSP"=w429, "nID"=0, "pSPT"=refnum<vi> refnum, "nWinType"=w424, "sIcon"=w422) -> (w430:T1)
          n202 = local write "tWindow_Out"(w430) -> ()
        }
      }
    }
  }
